vi "Check Status.vi"(8 "error in (no error)":errorcluster, 11 "Two Lockins in":refnum<class "Two Lockins.lvclass">) -> (0 "error out":errorcluster, 1 "Status":string, 2 "Ready?":bool, 3 "Two Lockins out":refnum<class "Two Lockins.lvclass">)   [LabVIEW 2017, in "Two Lockins.lvclass"]
doc: "(Dynamic) Check if the instrument is powered on and update its member fields with the instrument's current status. Optionally return a text status message."
uses:
  Two Lockins.lvclass
  Two Lockins.lvclass/Two Lockins.ctl
  Utility Classes/Readable/Readable.lvclass
  Lockin/sr830/SR830.lvlib
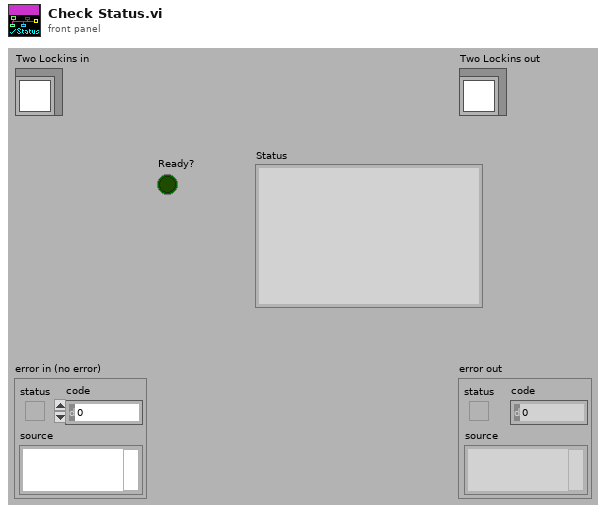
[diagram p1: front panel]
types:
  T1 = typedef "SR830.lvlib/Sensitivity_in_library.ctl" = u16
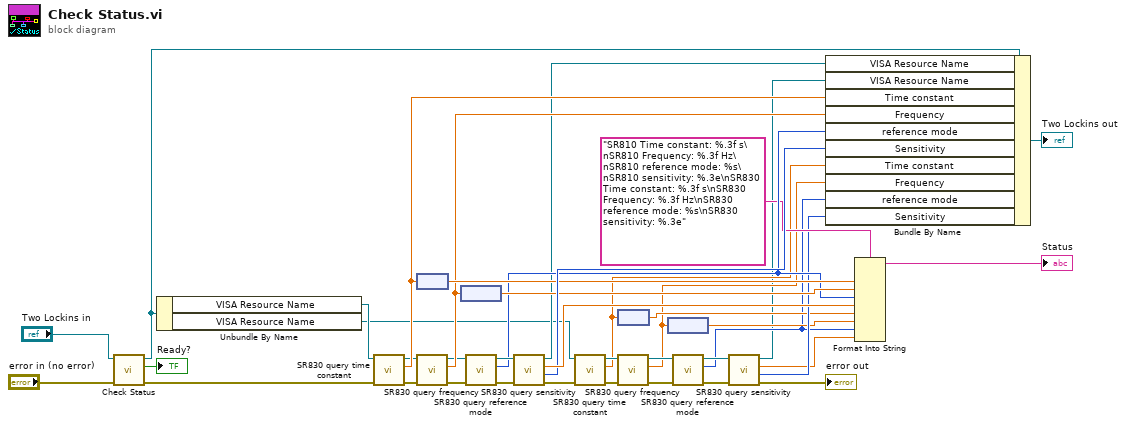
[diagram p0: block diagram]
diagram:
  n1 = call-parent "Check Status.vi"("error in (no error)"="error in (no error)", "Instrument in"="Two Lockins in") -> ("error out"=w6:errorcluster, "Ready?"=→"Ready?":bool, "Instrument out"=w16:refnum<class "Two Lockins.lvclass">)  [unwired: 6 in, 1 out]
  n2 = Unbundle By Name(w16) -> ("VISA Resource Name"=w2:refnum<visa-resource-name>, "VISA Resource Name"=w1:refnum<visa-resource-name>)
  n3 = call "SR830 query time constant.vi"("error in (no error)"=w6, "VISA resource name"=w2) -> ("error out"=w26:errorcluster, "time constant"=w29:dbl[unit], "VISA resource name out"=w24:refnum<visa-resource-name>)  [unwired: 7 in]
  n4 = node(w29) -> (w32:dbl)
  n5 = call "SR830 query frequency.vi"("error in (no error)"=w26, "VISA resource name"=w24) -> ("error out"=w27:errorcluster, "frequency"=w30:dbl[unit], "VISA resource name out"=w25:refnum<visa-resource-name>)  [unwired: 7 in]
  n6 = node(w30) -> (w33:dbl)
  n7 = call "SR830 query reference mode.vi"("error in (no error)"=w27, "VISA resource name"=w25) -> ("error out"=w35:errorcluster, "reference mode"=w31:enum16{"external", "internal"}, "VISA resource name out"=w34:refnum<visa-resource-name>)  [unwired: 7 in]
  n8 = call "SR830 query sensitivity.vi"("error in (no error)"=w35, "VISA resource name"=w34) -> ("error out"=w17:errorcluster, "Sensitivity"=w36:T1, "sensitivity"=w37:dbl[unit], "VISA resource name out"=w5:refnum<visa-resource-name>)  [unwired: 6 in]
  n9 = call "SR830 query time constant.vi"("error in (no error)"=w17, "VISA resource name"=w1) -> ("error out"=w21:errorcluster, "time constant"=w14:dbl[unit], "VISA resource name out"=w23:refnum<visa-resource-name>)  [unwired: 7 in]
  n10 = node(w14) -> (w13:dbl)
  n11 = call "SR830 query frequency.vi"("error in (no error)"=w21, "VISA resource name"=w23) -> ("error out"=w20:errorcluster, "frequency"=w12:dbl[unit], "VISA resource name out"=w22:refnum<visa-resource-name>)  [unwired: 7 in]
  n12 = node(w12) -> (w11:dbl)
  n13 = call "SR830 query reference mode.vi"("error in (no error)"=w20, "VISA resource name"=w22) -> ("error out"=w18:errorcluster, "reference mode"=w10:enum16{"external", "internal"}, "VISA resource name out"=w19:refnum<visa-resource-name>)  [unwired: 7 in]
  n14 = call "SR830 query sensitivity.vi"("error in (no error)"=w18, "VISA resource name"=w19) -> ("error out"=→"error out":errorcluster, "Sensitivity"=w15:T1, "sensitivity"=w9:dbl[unit], "VISA resource name out"=w4:refnum<visa-resource-name>)  [unwired: 6 in]
  n15 = Bundle By Name(cluster=w16, "VISA Resource Name"=w5, "VISA Resource Name"=w4, "Time constant"=w29, "Frequency"=w30, "reference mode"=w31, "Sensitivity"=w36, "Time constant"=w14, "Frequency"=w12, "reference mode"=w10, "Sensitivity"=w15) -> (→"Two Lockins out":refnum<class "Two Lockins.lvclass">)
  n16 = Format Into String(format string="SR810 Time constant: %.3f s\nSR810 Frequency: %.3f Hz\nSR810 reference mode: %s\nSR810 sensitivity: %.3e\nSR830 Time constant: %.3f s\nSR830 Frequency: %.3f Hz\nSR830 reference mode: %s\nSR830 sensitivity: %.3e", w32, w33, w31, w37, w13, w11, w10, w9) -> (resulting string=→"Status":string)  [unwired: 2 in, 1 out]
